vi "Fetch Single Record Multiple Channel(I16).vi"(5 "FIFO Type":enum16{"FPGA to Host FIFO (U64)", "Generic"}(ring), 7 "Timeout (s)":i32=5, 8 "error in":errorcluster, 11 "FPGA VI Reference In":refnum<k20>) -> (0 "error out":errorcluster, 2 "Acquired Data":i16[][](array[numeric]), 3 "FPGA VI Reference Out":refnum<k20>)   [LabVIEW 2012]
uses:
  <userlib>/FlexRIO Host Library/FlexRIO Host API/Acquire/Fetch/Fetch Acquired Data (U64).vi
  <vilib>/Utility/error.llb/Error Cluster From Error Code.vi
  <vilib>/rvi/errors/niLvFpgaAdjustHostInterfaceError.vi
  <vilib>/rvi/interface/nirviReadWriteControl/nirviReadWriteControl.xnode
  <userlib>/FlexRIO Host Library/FlexRIO Host Library (User).lvlib
  NiFpgaLv.dll
  <vilib>/rvi/interface/Simulation/niFpgaSimulationCallBeginRW.vi
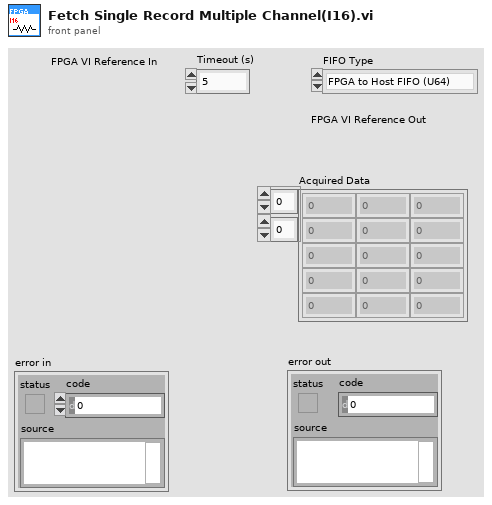
[diagram p1: front panel]
types:
  T1 = cluster{"Load Record Parameters?":bool, "Pre Trigger Samples":u16, "Samples per Record":u16, "Trigger Hold Off":u16, "Record Count":u16}
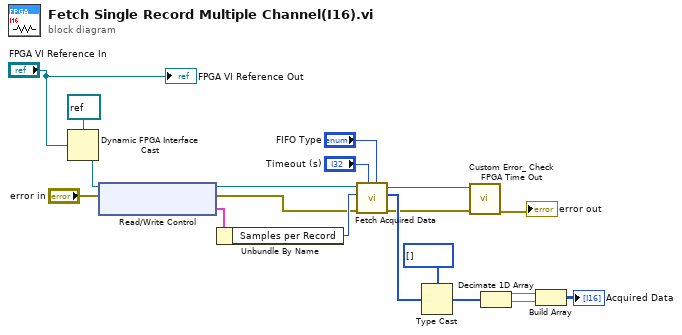
[diagram p0: block diagram]
diagram:
  n1 = Dynamic FPGA Interface Cast(Session In=refnum<k20> refnum ("Type"), Type="FPGA VI Reference In") -> (Session Out=w16:refnum<k20>)
  n2 = xnode "Read/Write Control"("FPGA VI Reference In"=w16, "error in"="error in") -> ("FPGA VI Reference Out"=w13:refnum<k20>, "error out"=w12:errorcluster, "Record Parameters"=w15:T1)
  n3 = Unbundle By Name(w15) -> ("Samples per Record"=w14:u16)
  n4 = call-poly <userlib>:"Fetch Acquired Data.vi"("FIFO Type"="FIFO Type", "Timeout (s)"="Timeout (s)", "error out"=w12, "Samples"=w14, "FPGA Reference In"=w13) -> ("error out"=w2:errorcluster, "Data"=w7:u64[], "FPGA Reference Out"=w3:refnum<k20>)  [unwired: 3 in, 1 out]
  n5 = Type Cast(type=i16[] [], x=w7) -> (*(type *) &x=w10:i16[])
  n6 = call <userlib>:"Custom Error_ Check FPGA Time Out.vi"("error in"=w2, "FPGA VI Reference In"=w3) -> ("error out"=→"error out":errorcluster)  [unwired: 8 in, 1 out]
  n7 = Decimate 1D Array(w10) -> (w9:i16[], w8:i16[])
  n8 = Build Array(w9, w8) -> (→"Acquired Data":i16[][])
  "FPGA VI Reference Out" <- "FPGA VI Reference In"
